vi "自动测试类型1.vi"(10 "测试类型1选择?":bool) -> ()   [LabVIEW 2010]
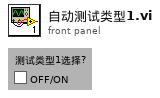
[diagram p1: front panel]
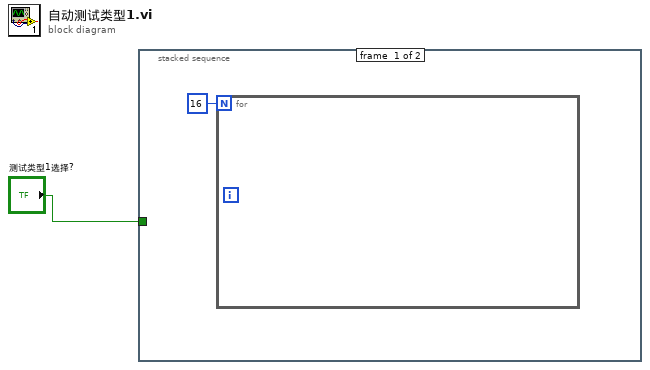
[diagram p0: block diagram]
diagram:
  n1 = stacked-sequence {
    tunnel: "测试类型1选择?" -> [_ w3]
    frame #0 {
      n2 = for {
        N: 16 -> [_]
      }
    }
    frame #1 {
      # "测试类型1统计结果"
      n3 = case shown="真" w3 {
        frame False {
        }
        frame True {
        }
      }
    }
  }
